vi "Format SQL COPY.vi"(6 "CSV?":bool=TRUE, 8 "error in (no error)":errorcluster, 10 "column name(s)":string, 11 "table name":string) -> (0 "error out":errorcluster, 3 "COPY SQL":string)   [LabVIEW 2016, in "PQ Connection.lvclass"]
uses:
  PQ Connection.lvclass
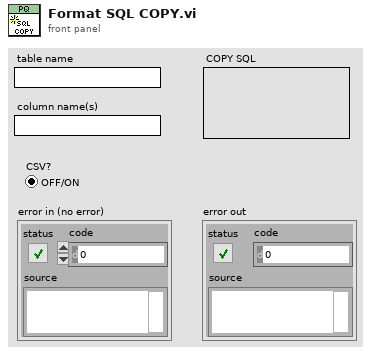
[diagram p1: front panel]
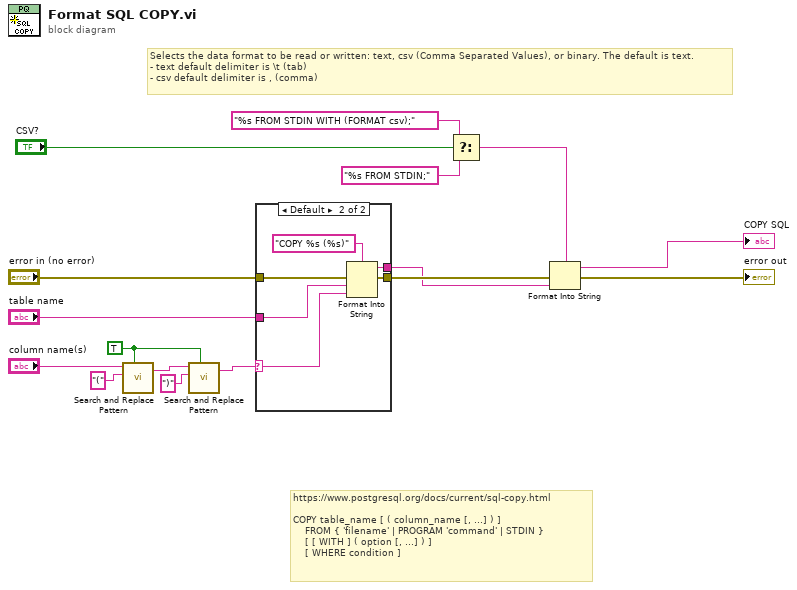
[diagram p0: block diagram]
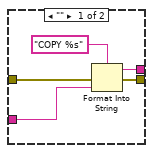
[diagram p2: hidden frame]
diagram:
  w5 = TRUE ("replace all? (F)")
  # "Selects the data format to be read or written: text, csv (Comma Separated Values), or binary. The default is text.\n- text default delimiter is \\t (tab)\n- csv default delimiter is , (comma)"
  # "https://www.postgresql.org/docs/current/sql-copy.html\n\nCOPY table_name [ ( column_name [, ...] ) ]\n    FROM { 'filename' | PROGRAM 'command' | STDIN }\n    [ [ WITH ] ( option [, ...] ) ]\n    [ WHERE condition ]"
  n1 = call <vilib>:"Search and Replace Pattern.vi"("string"="column name(s)", "regular expression (\"\")"="(" ("regular expression (\"\")"), "replace all? (F)"=w5) -> ("result string"=w3:string)  [unwired: 2 in, 1 out]
  n2 = call <vilib>:"Search and Replace Pattern.vi"("string"=w3, "regular expression (\"\")"=")" ("regular expression (\"\")"), "replace all? (F)"=w5) -> ("result string"=w4:string)  [unwired: 2 in, 1 out]
  n3 = case shown="Default" w4 {
    selector: w4 -> [_ w22]
    tunnel: "table name" -> [w21 w27]
    tunnel: [w20 w26] -> w10
    tunnel: "error in (no error)" -> [w18 w23]
    tunnel: [w17 w24] -> w14
    frame "" {
      n4 = Format Into String(format string="COPY %s" ("command"), error in=w18, w21) -> (resulting string=w20:string, error out=w17:errorcluster)  [unwired: 1 in]
    }
    frame Default {
      n5 = Format Into String(format string="COPY %s (%s)" ("command"), error in=w23, w27, w22) -> (resulting string=w26:string, error out=w24:errorcluster)  [unwired: 1 in]
    }
  }
  n6 = Select(t="%s FROM STDIN WITH (FORMAT csv);" ("command"), s="CSV?", f="%s FROM STDIN;" ("command")) -> (s? t:f=w12:string)
  n7 = Format Into String(format string=w12, error in=w14, w10) -> (resulting string=→"COPY SQL":string, error out=→"error out":errorcluster)  [unwired: 1 in]
